vi "close_sessions.vi"(4 "session bundle in":T1={"relay session out"={"VISA resource out"="COM12", "error out"={"status"=FALSE, "code"=0, "source"=""}}, "kloehn session out"={"VISA resource out"="COM12", "error out"={"status"=FALSE, "code"=0, "source"=""}}, "LiCor session out"={"VISA resource out"="COM12", "error out"={"status"=FALSE, "code"=0, "source"=""}}}) -> (0 "LiCor error out":errorcluster, 1 "kloehn error out":errorcluster, 2 "relay error out":errorcluster)   [LabVIEW 2010]
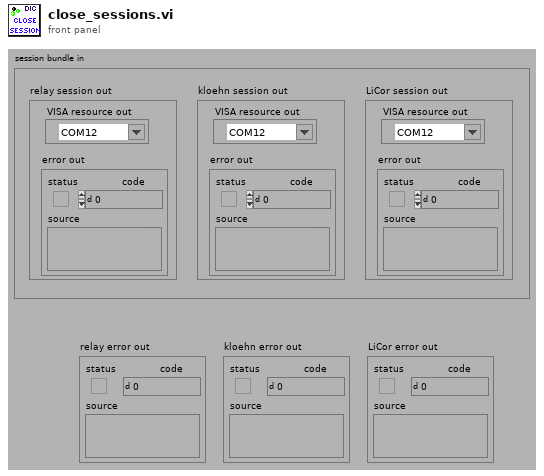
[diagram p1: front panel]
types:
  T1 = cluster{"relay session out":cluster{"VISA resource out":refnum<visa-resource-name>, "error out":errorcluster}, "kloehn session out":cluster{"VISA resource out":refnum<visa-resource-name>, "error out":errorcluster}, "LiCor session out":cluster{"VISA resource out":refnum<visa-resource-name>, "error out":errorcluster}}
  T2 = cluster{"VISA resource out":refnum<visa-resource-name>, "error out":errorcluster}
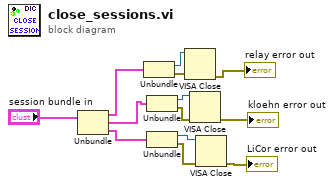
[diagram p0: block diagram]
diagram:
  n1 = Unbundle("session bundle in") -> ("relay session out"=w6:T2, "kloehn session out"=w5:T2, "LiCor session out"=w4:T2)
  n2 = Unbundle(w6) -> ("VISA resource out"=w12:refnum<visa-resource-name>, "error out"=w11:errorcluster)
  n3 = Unbundle(w5) -> ("VISA resource out"=w10:refnum<visa-resource-name>, "error out"=w9:errorcluster)
  n4 = Unbundle(w4) -> ("VISA resource out"=w8:refnum<visa-resource-name>, "error out"=w7:errorcluster)
  n5 = VISA Close(VISA resource name=w12, error in (no error)=w11) -> (error out=→"relay error out":errorcluster)
  n6 = VISA Close(VISA resource name=w10, error in (no error)=w9) -> (error out=→"kloehn error out":errorcluster)
  n7 = VISA Close(VISA resource name=w8, error in (no error)=w7) -> (error out=→"LiCor error out":errorcluster)
